vi "SVXMPL_Data to Process.vi"(0 "acquisition task":T1={"AI device settings"={"AI device"=0, "AI taskID"=0, "response"=[]}, "acquisition type"=enum."Finite", "measurement settings"={"AI sampling frequency"=0.0, "AO sampling frequency"=0.0, "AI block size"=0, "AO block Size"=0, "block duration [ms]"=0.0, "number of AI channels"=0, "board propagation time [samples]"=0, "DUT propagation time [s]"=0.0}, "settling settings"={"settle time"=0.015599999576807022, "settle cycles"=5}, "integration settings"={"integration time"=0.015599999576807022, "integration cycles"=5}, "AO device settings"={"AO device"=1, "AO taskID"=0, "excitation"=[]}, "acquisition accounting"={"initial read size [samples]"=0, "read offset [samples]"=0, "read length [samples]"=0, "blocks to settle [samples]"=0, "min delay until transition [samples]"=0}, "frequency range"={"start frequency"=0.0, "stop frequency"=0.0}, "block type"=enum."Initialize", "source settings"={"signal type"=enum."Sine wave", "frequency"=0.0, "total amplitude"=0.0, "frequencies"=[1.0], "relative amplitudes"=[1.0], "offset"=1.0, "total amplitude list"=[1.0], "ramping rate"=0.0}} {"source settings"."total amplitude" format="%.2f"; "source settings"."relative amplitudes" format="%.2f"; "source settings"."frequencies" format="%.2f"; "source settings"."total amplitude list" format="%.2f"; "source settings"."ramping rate" format="%.4f"; "source settings"."offset" format="%.2f"; "source settings"."frequency" format="%.2f"; "frequency range"."stop frequency" format="%.2f"; "frequency range"."start frequency" format="%.2f"; "AO device settings"."excitation"."output limits"."low limit (-10 V)" format="%.2f"; "AO device settings"."excitation"."output limits"."high limit (10 V)" format="%.2f"; "AI device settings"."response"."input limits"."low limit (0.0)" format="%.2f"; "AI device settings"."response"."input limits"."high limit (0.0)" format="%.2f"; "integration settings"."integration time" format="%.2p"; "settling settings"."settle time" format="%.2p"; "measurement settings"."DUT propagation time [s]" format="%.2f"; "measurement settings"."AO sampling frequency" format="%.2f"; "measurement settings"."AI sampling frequency" format="%.2f"}, 5 "waveform data":waveform(dbl)[](array[waveform]), 11 "error in (no error)":errorcluster) -> (4 "dup acquisition task":T1={"AI device settings"={"AI device"=0, "AI taskID"=0, "response"=[]}, "acquisition type"=enum."Finite", "measurement settings"={"AI sampling frequency"=0.0, "AO sampling frequency"=0.0, "AI block size"=0, "AO block Size"=0, "block duration [ms]"=0.0, "number of AI channels"=0, "board propagation time [samples]"=0, "DUT propagation time [s]"=0.0}, "settling settings"={"settle time"=0.015599999576807022, "settle cycles"=5}, "integration settings"={"integration time"=0.015599999576807022, "integration cycles"=5}, "AO device settings"={"AO device"=1, "AO taskID"=0, "excitation"=[]}, "acquisition accounting"={"initial read size [samples]"=0, "read offset [samples]"=0, "read length [samples]"=0, "blocks to settle [samples]"=0, "min delay until transition [samples]"=0}, "frequency range"={"start frequency"=0.0, "stop frequency"=0.0}, "block type"=enum."Initialize", "source settings"={"signal type"=enum."Sine wave", "frequency"=0.0, "total amplitude"=0.0, "frequencies"=[1.0], "relative amplitudes"=[1.0], "offset"=1.0, "total amplitude list"=[1.0], "ramping rate"=0.0}} {"source settings"."total amplitude" format="%.2f"; "source settings"."relative amplitudes" format="%.2f"; "source settings"."frequencies" format="%.2f"; "source settings"."total amplitude list" format="%.2f"; "source settings"."ramping rate" format="%.4f"; "source settings"."offset" format="%.2f"; "source settings"."frequency" format="%.2f"; "frequency range"."stop frequency" format="%.2f"; "frequency range"."start frequency" format="%.2f"; "AO device settings"."excitation"."output limits"."low limit (-10 V)" format="%.2f"; "AO device settings"."excitation"."output limits"."high limit (10 V)" format="%.2f"; "AI device settings"."response"."input limits"."low limit (0.0)" format="%.2f"; "AI device settings"."response"."input limits"."high limit (0.0)" format="%.2f"; "integration settings"."integration time" format="%.2p"; "settling settings"."settle time" format="%.2p"; "measurement settings"."DUT propagation time [s]" format="%.2f"; "measurement settings"."AO sampling frequency" format="%.2f"; "measurement settings"."AI sampling frequency" format="%.2f"}, 6 "data to process":waveform(dbl)[](array[waveform]), 8 "new data to process":bool, 15 "error out":errorcluster)   [LabVIEW 2017]
uses:
  <vilib>/addons/Sound and Vibration/compatibility/Example Support/SVXMPL_Acquisition Task.ctl
  <vilib>/Waveform/WDTOps.llb/WDT Get Waveform Subset DBL (LV80).vi
panel:
  in  "empty":waveform(dbl)[](array[waveform])
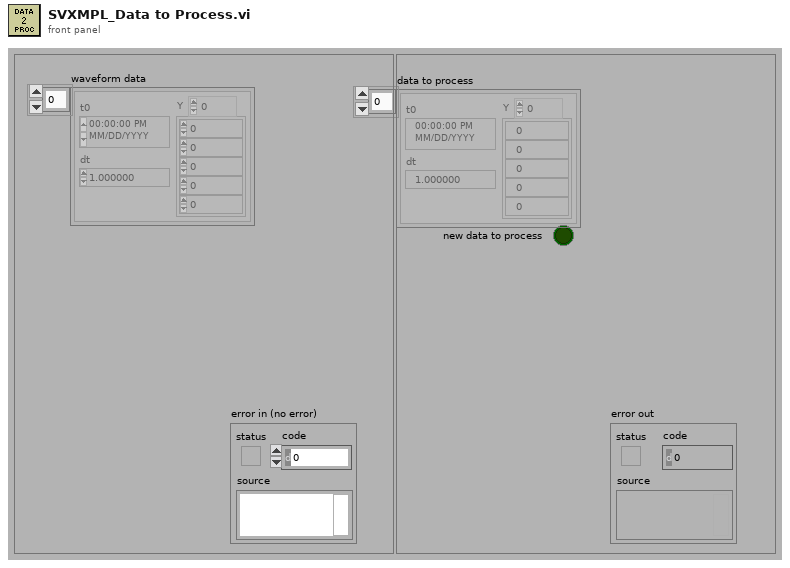
[diagram p1: front panel]
types:
  T1 = typedef "SVXMPL_Acquisition Task.ctl" = cluster{"AI device settings":cluster{"AI device":i16, "AI taskID":u32, "response":cluster{"AI channel":tag, "input limits":cluster{"high limit (0.0)":sgl, "low limit (0.0)":sgl}, "coupling & input config":cluster{"coupling":enum16{"no change", "DC", "AC", "GND", "internal ref."}, "input config":enum16{"no change", "differential", "ref. single-ended", "non-ref. single-ended", "4-wire"}}}[]}, "acquisition type":enum16{"Finite", "Averaged", "Settled", "Amplitude Sweep"}, "measurement settings":cluster{"AI sampling frequency":dbl, "AO sampling frequency":dbl, "AI block size":i32, "AO block Size":i32, "block duration [ms]":dbl, "number of AI channels":i32, "board propagation time [samples]":i32, "DUT propagation time [s]":dbl}, "settling settings":cluster{"settle time":dbl, "settle cycles":i32}, "integration settings":cluster{"integration time":dbl, "integration cycles":i32}, "AO device settings":cluster{"AO device":i16, "AO taskID":u32, "excitation":cluster{"AO Channel":tag, "output limits":cluster{"high limit (10 V)":sgl, "low limit (-10 V)":sgl, "reference source":enum16{"no change", "internal", "external"}}}[]}, "acquisition accounting":cluster{"initial read size [samples]":i32, "read offset [samples]":i32, "read length [samples]":i32, "blocks to settle [samples]":i32, "min delay until transition [samples]":i32}, "frequency range":cluster{"start frequency":dbl, "stop frequency":dbl}, "block type":enum16{"Initialize", "Settle", "Integrate"}, "source settings":cluster{"signal type":enum16{"Sine wave", "Dual tone (IMD)", "Multitone", "Chirp", "Frequency flat chirp", "Uniform white noise", "Gaussian white noise", "Pink noise", "PRN"}, "frequency":dbl, "total amplitude":dbl, "frequencies":dbl[], "relative amplitudes":dbl[], "offset":dbl, "total amplitude list":dbl[], "ramping rate":dbl}}
  T2 = enum16{"Finite", "Averaged", "Settled", "Amplitude Sweep"}
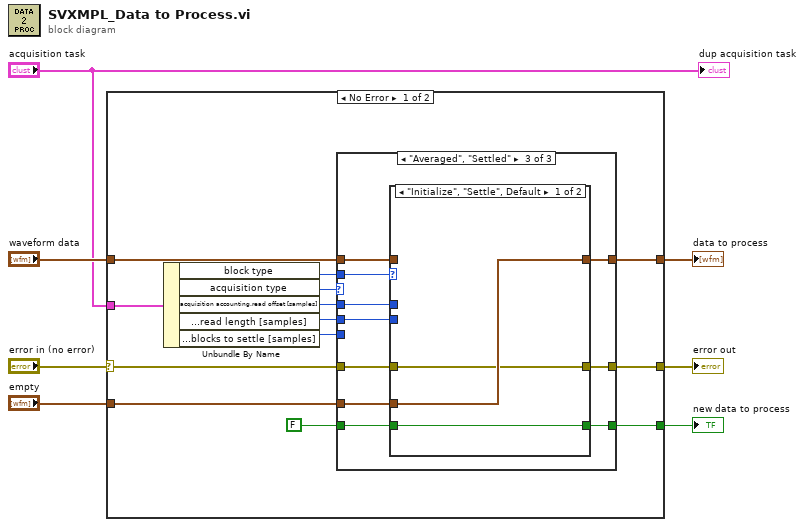
[diagram p0: block diagram]
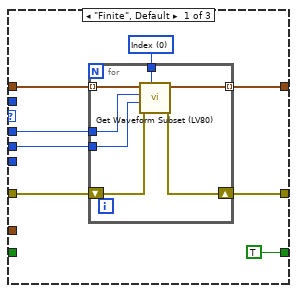
[diagram p2: hidden frame]
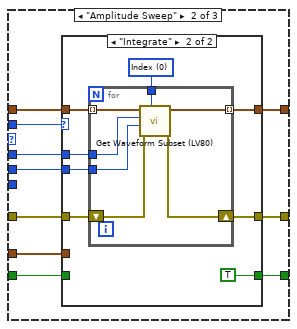
[diagram p3: hidden frame]
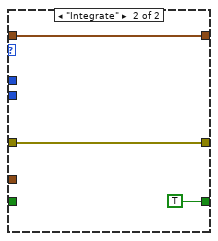
[diagram p5: hidden frame]
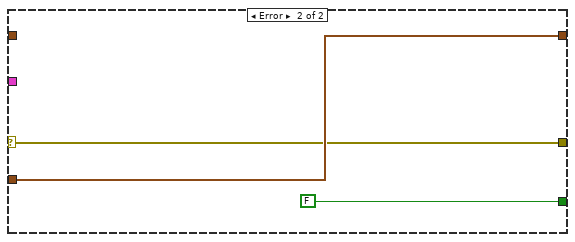
[diagram p6: hidden frame]
diagram:
  n1 = case shown="No Error" "error in (no error)" {
    selector: "error in (no error)" -> [w9 w80]
    tunnel: "acquisition task" -> [w20 _]
    tunnel: [w18 FALSE ("Boolean")] -> w7
    tunnel: "empty" -> [w16 w82]
    tunnel: [w15 w82] -> w5
    tunnel: "waveform data" -> [w14 _]
    tunnel: [w8 w80] -> w2
    frame No Error {
      n2 = Unbundle By Name(w20) -> ("block type"=w19:enum16{"Initialize", "Settle", "Integrate"}, "acquisition type"=w10:T2, "acquisition accounting.read offset [samples]"=w11:i32, "acquisition accounting.read length [samples]"=w12:i32, "acquisition accounting.blocks to settle [samples]"=w13:i32)
      n3 = case shown="\"Averaged\", \"Settled\"" w10 {
        tunnel: w11 -> [w25 w43 w71]
        tunnel: w12 -> [w24 w42 w70]
        tunnel: w13 -> [_ _ _]
        tunnel: w14 -> [w28 w45 w73]
        tunnel: [w27 w44 w72] -> w15
        tunnel: w16 -> [_ w41 w69]
        tunnel: FALSE ("Boolean") -> [_ w40 w68]
        tunnel: [TRUE w39 w67] -> w18
        tunnel: w19 -> [_ w38 w66]
        tunnel: w9 -> [w21 w37 w65]
        tunnel: [w22 w36 w64] -> w8
        frame "Finite", Default {
          w26 = u16 0 items=["Index", "Relative Time"] ("Mode")
          n4 = for {
            tunnel: w28 -> [w35] mode=indexing
            tunnel: w26 -> [w34]
            tunnel: [w33] -> w27 mode=indexing
            tunnel: w25 -> [w32]
            tunnel: w24 -> [w31]
            shift-right: [w30] -> w22
            shift-left: w21 -> [w29]
            n5 = call-poly <vilib>:"Get Waveform Subset (LV80).vi"("start/duration format"=w34, "error in (no error)"=w29, "duration"=w31, "start samples/time"=w32, "waveform in"=w35) -> ("error out"=w30:errorcluster, "waveform out"=w33:waveform(dbl))  [unwired: 1 in, 2 out]
          }
        }
        frame "Amplitude Sweep" {
          n6 = case shown="\"Integrate\"" w38 {
            tunnel: w45 -> [_ w56]
            tunnel: [w48 w55] -> w44
            tunnel: w43 -> [_ w53]
            tunnel: w42 -> [_ w52]
            tunnel: w41 -> [w48 _]
            tunnel: w40 -> [w47 _]
            tunnel: [w47 TRUE] -> w39
            tunnel: w37 -> [w46 w50]
            tunnel: [w46 w49] -> w36
            frame "Initialize", Default {
            }
            frame "Integrate" {
              w54 = u16 0 items=["Index", "Relative Time"] ("Mode")
              n7 = for {
                tunnel: w56 -> [w63] mode=indexing
                tunnel: w54 -> [w62]
                tunnel: [w61] -> w55 mode=indexing
                tunnel: w53 -> [w60]
                tunnel: w52 -> [w59]
                shift-right: [w57] -> w49
                shift-left: w50 -> [w58]
                n8 = call-poly <vilib>:"Get Waveform Subset (LV80).vi"("start/duration format"=w62, "error in (no error)"=w58, "duration"=w59, "start samples/time"=w60, "waveform in"=w63) -> ("error out"=w57:errorcluster, "waveform out"=w61:waveform(dbl))  [unwired: 1 in, 2 out]
              }
            }
          }
        }
        frame "Averaged", "Settled" {
          n9 = case shown="\"Initialize\", \"Settle\", Default" w66 {
            tunnel: w73 -> [_ w77]
            tunnel: [w76 w77] -> w72
            tunnel: w71 -> [_ _]
            tunnel: w70 -> [_ _]
            tunnel: w69 -> [w76 _]
            tunnel: w68 -> [w75 _]
            tunnel: [w75 TRUE] -> w67
            tunnel: w65 -> [w74 w78]
            tunnel: [w74 w78] -> w64
            frame "Initialize", "Settle", Default {
            }
            frame "Integrate" {
            }
          }
        }
      }
    }
    frame Error {
    }
  }
  "new data to process" <- w7
  "data to process" <- w5
  "error out" <- w2
  "dup acquisition task" <- "acquisition task"
